vi "Get Attribute DBL.vi"(8 "error in":errorcluster, 10 "Attribute":string, 11 "ConfigFromJSON in":refnum<class "Config from JSON.lvclass">) -> (0 "error out":errorcluster, 2 "Value":dbl, 3 "ConfigFromJSON out":refnum<class "Config from JSON.lvclass">)   [LabVIEW 2024, in "Config from JSON.lvclass"]
uses:
  Config from JSON.lvclass
  Config from JSON.lvclass/Config from JSON.ctl
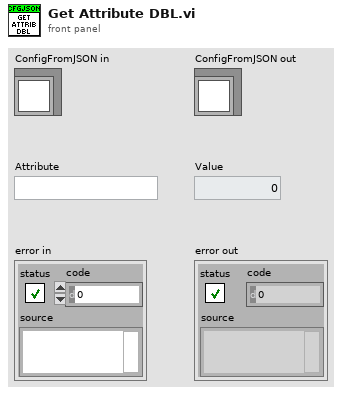
[diagram p1: front panel]
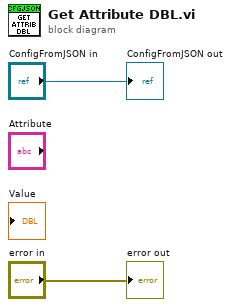
[diagram p0: block diagram]
diagram:
  "error out" <- "error in"
  "ConfigFromJSON out" <- "ConfigFromJSON in"
